vi "写入点.vi"(8 "error in (no error)":errorcluster caption="错误输入（无错误）", 10 "点":T1 caption="点（双精度）", 11 "点输入":refnum<class "点.lvclass">) -> (0 "error out":errorcluster caption="错误输出", 3 "点输出":refnum<class "点.lvclass">)   [LabVIEW 2011, in "点.lvclass"]
uses:
  <vilib>/Utility/miscctls.llb/LVPointDoubleTypeDef.ctl
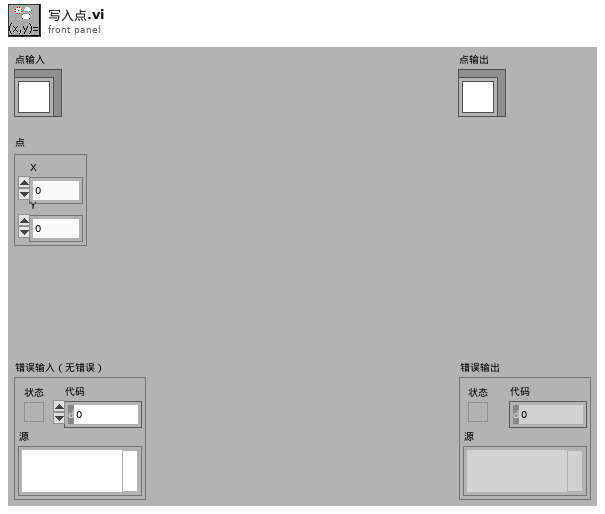
[diagram p1: front panel]
types:
  T1 = typedef "LVPointDoubleTypeDef.ctl" = cluster{"X":dbl, "Y":dbl}
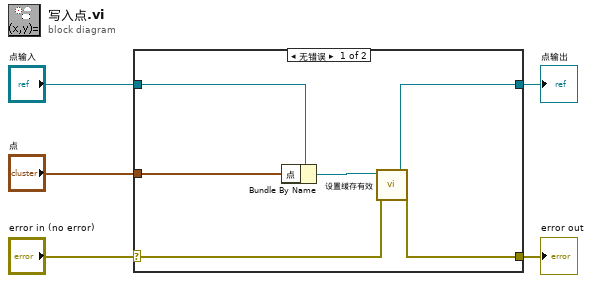
[diagram p0: block diagram]
diagram:
  n1 = case shown="无错误" "error in (no error)" {
    selector: "error in (no error)" -> [w7 w12]
    tunnel: [w6 w12] -> w4
    tunnel: [w8 w13] -> w2
    tunnel: "点输入" -> [w11 w13]
    tunnel: "点" -> [w10 _]
    frame No Error {
      n2 = Bundle By Name(cluster=w11, "点"=w10) -> (w9:refnum<class "点.lvclass">)
      n3 = call "设置缓存有效.vi"("error in (no error)"=w7, "图形 输入"=w9) -> ("error out"=w6:errorcluster, "图形 输出"=w8:refnum<class "点.lvclass">)  [unwired: 8 in]
    }
    frame Error {
    }
  }
  "error out" <- w4
  "点输出" <- w2
